vi "Set End Point.vi"(8 "error in (no error)":errorcluster, 9 "point":cluster{"x":i16, "y":i16}, 10 "End":enum16{"Source", "Target"}(ring), 11 "FSM.Edge in":refnum<class "FSM.Edge.lvclass">) -> (0 "error out":errorcluster, 3 "FSM.Edge out":refnum<class "FSM.Edge.lvclass">)   [LabVIEW 2015, in "FSM.Edge.lvclass"]
uses:
  FSM.Edge.lvclass
  FSM.Edge.lvclass/FSM.Edge.ctl
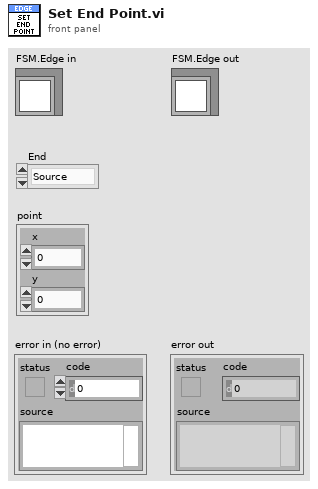
[diagram p1: front panel]
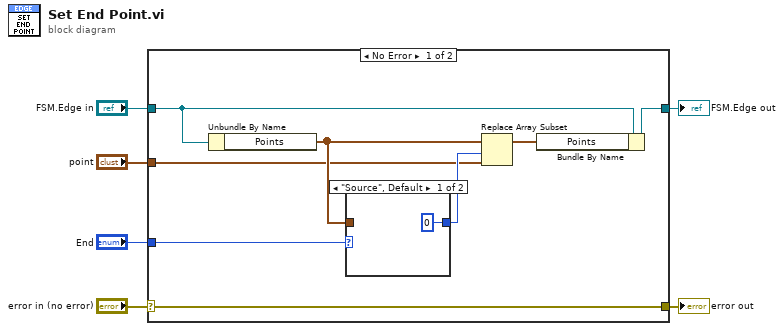
[diagram p0: block diagram]
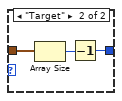
[diagram p2: hidden frame]
diagram:
  n1 = case shown="No Error" "error in (no error)" {
    selector: "error in (no error)" -> [w14 w20]
    tunnel: [w14 w20] -> w5
    tunnel: [w8 w19] -> w3
    tunnel: "FSM.Edge in" -> [w13 w19]
    tunnel: "End" -> [w12 _]
    tunnel: "point" -> [w9 _]
    frame No Error {
      n2 = Unbundle By Name(w13) -> ("Points"=w11:cluster{"x":i16, "y":i16}[])
      n3 = case shown="\"Source\", Default" w12 {
        tunnel: w11 -> [_ w18]
        tunnel: [0 w16] -> w10
        frame "Source", Default {
        }
        frame "Target" {
          n4 = Array Size(array=w18) -> (size(s)=w17:i32)
          n5 = Decrement(x=w17) -> (x-1=w16:i32)
        }
      }
      n6 = Replace Array Subset(array=w11, new element=w9, index=w10) -> (w7:cluster{"x":i16, "y":i16}[])
      n7 = Bundle By Name(cluster=w13, "Points"=w7) -> (w8:refnum<class "FSM.Edge.lvclass">)
    }
    frame Error {
    }
  }
  "error out" <- w5
  "FSM.Edge out" <- w3
